vi "easyUiMap.vi"() -> ()   [LabVIEW 2020]
panel:
  out "Schlüssel nicht gefunden?":bool
  out "Wert":i32
  out "Map":map{string, i32}(c390)
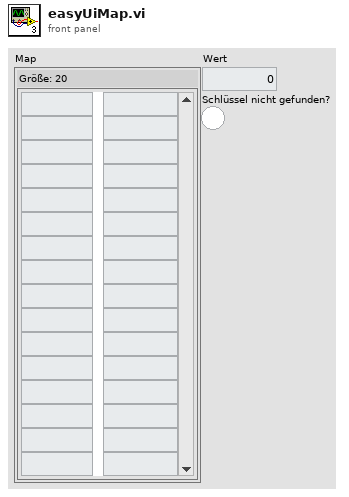
[diagram p1: front panel]
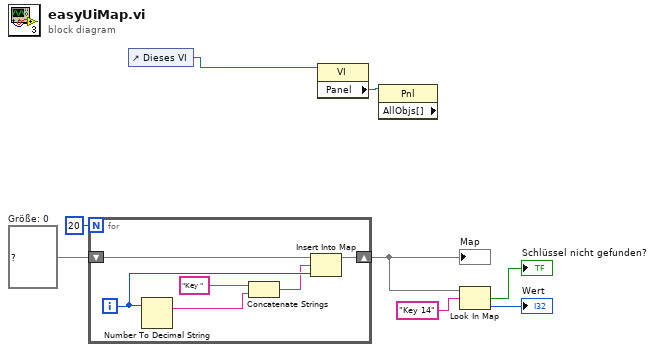
[diagram p0: block diagram]
diagram:
  w8 = map{string, i32} {}  # Größe: 0
  n1 = for {
    N: 20 -> [_]
    shift-right: [w13] -> w6
    shift-left: w8 -> [w14]
    i -> [w11]
    n2 = Number To Decimal String(number=w11) -> (decimal integer string=w9:string)  [unwired: 1 in]
    n3 = Concatenate Strings("Key ", w9) -> (w10:string)
    n4 = Insert Into Map(map in=w14, key=w10, value=w11) -> (map out=w13:map{string, i32})  [unwired: 2 out]
  }
  "Map" <- w6
  n5 = control-ref of="Dieses VI"() -> (w2:refnum<vi>)
  n6 = property class="VI"(reference=w2) -> ("Panel"=w1:refnum<vi>)  [unwired: 1 in, 2 out]
  n7 = property class="Pnl" props=["AllObjs[]"](reference=w1) -> ()  [unwired: 1 in, 3 out]
  n8 = Look In Map(map=w6, key="Key 14" ("Schlüssel")) -> (key not found?=→"Schlüssel nicht gefunden?":bool, value=→"Wert":i32)  [unwired: 1 in]
